vi "Deadband.vi"(9 "Input":dbl, 11 "Deadband":dbl) -> (2 "Output":dbl)   [LabVIEW 2012]
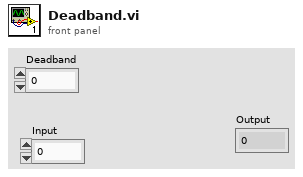
[diagram p1: front panel]
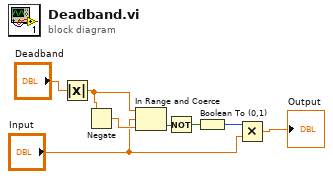
[diagram p0: block diagram]
diagram:
  n1 = Absolute Value(x="Deadband") -> (abs(x)=w7:dbl)
  n2 = Negate(x=w7) -> (-x=w6:dbl)
  n3 = In Range and Coerce(upper limit=w7, x="Input", lower limit=w6) -> (In Range?=w5:bool)  [unwired: 1 out]
  n4 = Not(x=w5) -> (.not. x?=w4:bool)
  n5 = Boolean To (0,1)(Boolean=w4) -> (0, 1=w3:i16)
  n6 = Multiply(x=w3, y="Input") -> (x*y=→"Output":dbl)
